vi "随机生成扑克牌.vi"() -> (0 "牌4值":dbl, 1 "牌2值":dbl, 2 "牌3值":dbl, 3 "牌1值":dbl, 4 "牌4":dbl, 5 "牌3":dbl, 6 "牌2":dbl, 7 "牌1":dbl)   [LabVIEW 2014]
panel:
  in  "布尔":bool
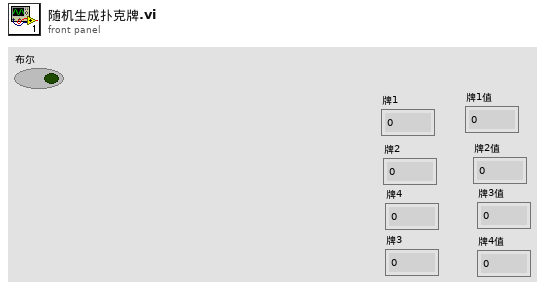
[diagram p1: front panel]
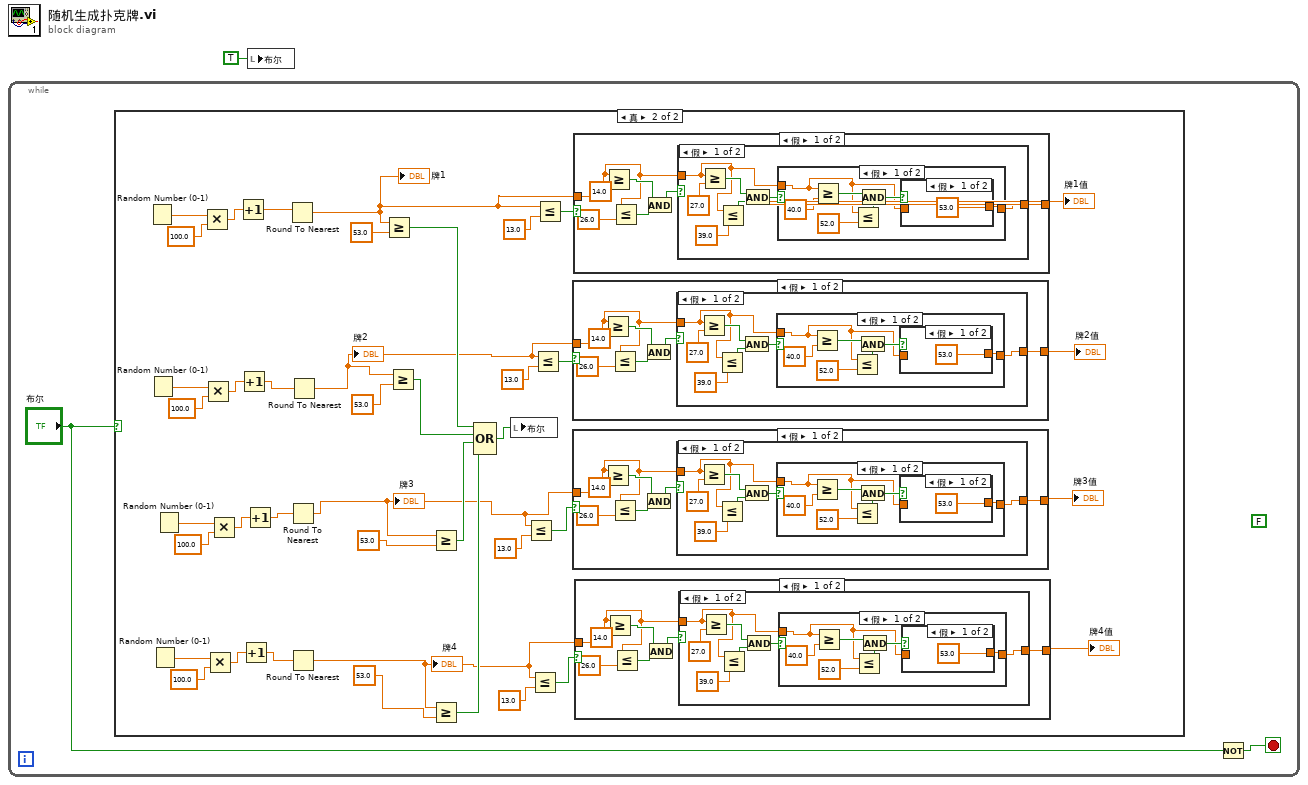
[diagram p0: block diagram]
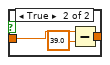
[diagram p3: hidden frame]
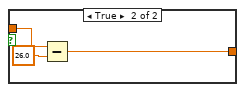
[diagram p4: hidden frame]
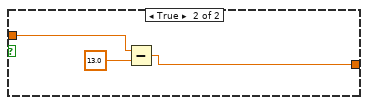
[diagram p5: hidden frame]
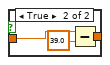
[diagram p7: hidden frame]
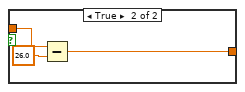
[diagram p8: hidden frame]
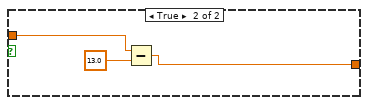
[diagram p9: hidden frame]
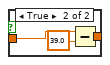
[diagram p11: hidden frame]
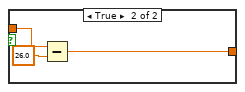
[diagram p12: hidden frame]
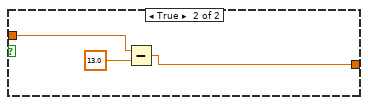
[diagram p13: hidden frame]
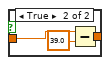
[diagram p15: hidden frame]
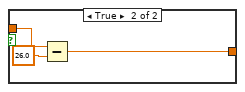
[diagram p16: hidden frame]
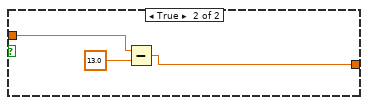
[diagram p17: hidden frame]
diagram:
  n1 = while {
    stop <- w3 stop-if-true
    (unwired) FALSE
    n2 = case shown="真" "布尔" {
      frame False {
      }
      frame True {
        n3 = Random Number (0-1)() -> (number: 0 to 1=w30:dbl)
        n4 = Random Number (0-1)() -> (number: 0 to 1=w27:dbl)
        n5 = Random Number (0-1)() -> (number: 0 to 1=w20:dbl)
        n6 = Random Number (0-1)() -> (number: 0 to 1=w23:dbl)
        n7 = Multiply(x=w30, y=100.0) -> (x*y=w29:dbl)
        n8 = Multiply(x=w27, y=100.0) -> (x*y=w28:dbl)
        n9 = Multiply(x=w20, y=100.0) -> (x*y=w21:dbl)
        n10 = Multiply(x=w23, y=100.0) -> (x*y=w22:dbl)
        n11 = Increment(x=w29) -> (x+1=w11:dbl)
        n12 = Increment(x=w28) -> (x+1=w5:dbl)
        n13 = Increment(x=w21) -> (x+1=w9:dbl)
        n14 = Increment(x=w22) -> (x+1=w7:dbl)
        n15 = Round To Nearest(number=w11) -> (nearest integer value=w10:dbl)
        "牌1" <- w10
        n16 = Round To Nearest(number=w7) -> (nearest integer value=w6:dbl)
        "牌3" <- w6
        n17 = Round To Nearest(number=w9) -> (nearest integer value=w8:dbl)
        "牌4" <- w8
        n18 = Round To Nearest(number=w5) -> (nearest integer value=w4:dbl)
        "牌2" <- w4
        n19 = Greater Or Equal?(x=w10, y=53.0) -> (x >= y?=w16:bool)
        n20 = Greater Or Equal?(x=w4, y=53.0) -> (x >= y?=w15:bool)
        n21 = Greater Or Equal?(x=w6, y=53.0) -> (x >= y?=w14:bool)
        n22 = Greater Or Equal?(x=w8, y=53.0) -> (x >= y?=w13:bool)
        n23 = Compound Arithmetic op=OR(w16, w15, w14, w13) -> (w12:bool)
        n24 = local write "布尔"(w12) -> ()
        n25 = Less Or Equal?(x=w6, y=13.0) -> (x <= y?=w34:bool)
        n26 = Less Or Equal?(x=w8, y=13.0) -> (x <= y?=w33:bool)
        n27 = Less Or Equal?(x=w4, y=13.0) -> (x <= y?=w35:bool)
        n28 = Less Or Equal?(x=w10, y=13.0) -> (x <= y?=w36:bool)
        n29 = case shown="假" w35 {
          tunnel: [w109 w140] -> w39
          tunnel: w4 -> [w110 w140]
          frame False {
            n30 = Greater Or Equal?(x=w110, y=14.0) -> (x >= y?=w112:bool)
            n31 = Less Or Equal?(x=w110, y=26.0) -> (x <= y?=w113:bool)
            n32 = And(x=w112, y=w113) -> (x .and. y?=w111:bool)
            n33 = case shown="假" w111 {
              tunnel: w110 -> [w117 w138]
              tunnel: [w116 w137] -> w109
              frame False {
                n34 = Greater Or Equal?(x=w117, y=27.0) -> (x >= y?=w120:bool)
                n35 = Less Or Equal?(x=w117, y=39.0) -> (x <= y?=w119:bool)
                n36 = And(x=w120, y=w119) -> (x .and. y?=w118:bool)
                n37 = case shown="假" w118 {
                  tunnel: w117 -> [w125 w136]
                  tunnel: [w124 w134] -> w116
                  frame False {
                    n38 = Greater Or Equal?(x=w125, y=40.0) -> (x >= y?=w127:bool)
                    n39 = Less Or Equal?(x=w125, y=52.0) -> (x <= y?=w123:bool)
                    n40 = And(x=w127, y=w123) -> (x .and. y?=w126:bool)
                    n41 = case shown="假" w126 {
                      tunnel: w125 -> [_ w132]
                      tunnel: [53.0 ("y") w131] -> w124
                      frame False {
                      }
                      frame True {
                        n42 = Subtract(x=w132, y=39.0) -> (x-y=w131:dbl)
                      }
                    }
                  }
                  frame True {
                    n43 = Subtract(x=w136, y=26.0) -> (x-y=w134:dbl)
                  }
                }
              }
              frame True {
                n44 = Subtract(x=w138, y=13.0) -> (x-y=w137:dbl)
              }
            }
          }
          frame True {
          }
        }
        "牌2值" <- w39
        n45 = case shown="假" w34 {
          tunnel: [w77 w108] -> w38
          tunnel: w6 -> [w78 w108]
          frame False {
            n46 = Greater Or Equal?(x=w78, y=14.0) -> (x >= y?=w80:bool)
            n47 = Less Or Equal?(x=w78, y=26.0) -> (x <= y?=w81:bool)
            n48 = And(x=w80, y=w81) -> (x .and. y?=w79:bool)
            n49 = case shown="假" w79 {
              tunnel: w78 -> [w85 w106]
              tunnel: [w84 w105] -> w77
              frame False {
                n50 = Greater Or Equal?(x=w85, y=27.0) -> (x >= y?=w88:bool)
                n51 = Less Or Equal?(x=w85, y=39.0) -> (x <= y?=w87:bool)
                n52 = And(x=w88, y=w87) -> (x .and. y?=w86:bool)
                n53 = case shown="假" w86 {
                  tunnel: w85 -> [w93 w104]
                  tunnel: [w92 w102] -> w84
                  frame False {
                    n54 = Greater Or Equal?(x=w93, y=40.0) -> (x >= y?=w95:bool)
                    n55 = Less Or Equal?(x=w93, y=52.0) -> (x <= y?=w91:bool)
                    n56 = And(x=w95, y=w91) -> (x .and. y?=w94:bool)
                    n57 = case shown="假" w94 {
                      tunnel: w93 -> [_ w100]
                      tunnel: [53.0 ("y") w99] -> w92
                      frame False {
                      }
                      frame True {
                        n58 = Subtract(x=w100, y=39.0) -> (x-y=w99:dbl)
                      }
                    }
                  }
                  frame True {
                    n59 = Subtract(x=w104, y=26.0) -> (x-y=w102:dbl)
                  }
                }
              }
              frame True {
                n60 = Subtract(x=w106, y=13.0) -> (x-y=w105:dbl)
              }
            }
          }
          frame True {
          }
        }
        "牌3值" <- w38
        n61 = case shown="假" w36 {
          tunnel: [w141 w172] -> w43
          tunnel: w10 -> [w142 w172]
          frame False {
            n62 = Greater Or Equal?(x=w142, y=14.0) -> (x >= y?=w144:bool)
            n63 = Less Or Equal?(x=w142, y=26.0) -> (x <= y?=w145:bool)
            n64 = And(x=w144, y=w145) -> (x .and. y?=w143:bool)
            n65 = case shown="假" w143 {
              tunnel: w142 -> [w149 w170]
              tunnel: [w148 w169] -> w141
              frame False {
                n66 = Greater Or Equal?(x=w149, y=27.0) -> (x >= y?=w152:bool)
                n67 = Less Or Equal?(x=w149, y=39.0) -> (x <= y?=w151:bool)
                n68 = And(x=w152, y=w151) -> (x .and. y?=w150:bool)
                n69 = case shown="假" w150 {
                  tunnel: w149 -> [w157 w168]
                  tunnel: [w156 w166] -> w148
                  frame False {
                    n70 = Greater Or Equal?(x=w157, y=40.0) -> (x >= y?=w159:bool)
                    n71 = Less Or Equal?(x=w157, y=52.0) -> (x <= y?=w155:bool)
                    n72 = And(x=w159, y=w155) -> (x .and. y?=w158:bool)
                    n73 = case shown="假" w158 {
                      tunnel: w157 -> [_ w164]
                      tunnel: [53.0 ("y") w163] -> w156
                      frame False {
                      }
                      frame True {
                        n74 = Subtract(x=w164, y=39.0) -> (x-y=w163:dbl)
                      }
                    }
                  }
                  frame True {
                    n75 = Subtract(x=w168, y=26.0) -> (x-y=w166:dbl)
                  }
                }
              }
              frame True {
                n76 = Subtract(x=w170, y=13.0) -> (x-y=w169:dbl)
              }
            }
          }
          frame True {
          }
        }
        "牌1值" <- w43
        n77 = case shown="假" w33 {
          tunnel: [w45 w76] -> w37
          tunnel: w8 -> [w46 w76]
          frame False {
            n78 = Greater Or Equal?(x=w46, y=14.0) -> (x >= y?=w48:bool)
            n79 = Less Or Equal?(x=w46, y=26.0) -> (x <= y?=w49:bool)
            n80 = And(x=w48, y=w49) -> (x .and. y?=w47:bool)
            n81 = case shown="假" w47 {
              tunnel: w46 -> [w53 w74]
              tunnel: [w52 w73] -> w45
              frame False {
                n82 = Greater Or Equal?(x=w53, y=27.0) -> (x >= y?=w56:bool)
                n83 = Less Or Equal?(x=w53, y=39.0) -> (x <= y?=w55:bool)
                n84 = And(x=w56, y=w55) -> (x .and. y?=w54:bool)
                n85 = case shown="假" w54 {
                  tunnel: w53 -> [w61 w72]
                  tunnel: [w60 w70] -> w52
                  frame False {
                    n86 = Greater Or Equal?(x=w61, y=40.0) -> (x >= y?=w63:bool)
                    n87 = Less Or Equal?(x=w61, y=52.0) -> (x <= y?=w59:bool)
                    n88 = And(x=w63, y=w59) -> (x .and. y?=w62:bool)
                    n89 = case shown="假" w62 {
                      tunnel: w61 -> [_ w68]
                      tunnel: [53.0 ("y") w67] -> w60
                      frame False {
                      }
                      frame True {
                        n90 = Subtract(x=w68, y=39.0) -> (x-y=w67:dbl)
                      }
                    }
                  }
                  frame True {
                    n91 = Subtract(x=w72, y=26.0) -> (x-y=w70:dbl)
                  }
                }
              }
              frame True {
                n92 = Subtract(x=w74, y=13.0) -> (x-y=w73:dbl)
              }
            }
          }
          frame True {
          }
        }
        "牌4值" <- w37
      }
    }
    n93 = Not(x="布尔") -> (.not. x?=w3:bool)
  }
  n94 = local write "布尔"(TRUE ("布尔")) -> ()
